vi "3 Totes Rotate.vi"() -> ()   [LabVIEW 2014]
panel:
  in  "Feet 4":dbl=6.0 format="%#_13g"
  in  "Degrees 2":dbl=45.0 format="%#_13g"
  in  "Feet 3":dbl=6.0 format="%#_13g"
  in  "Feet 2":dbl=6.0 format="%#_13g"
  in  "Degrees":dbl=45.0 format="%#_13g"
  in  "Feet":dbl=6.0 format="%#_13g"
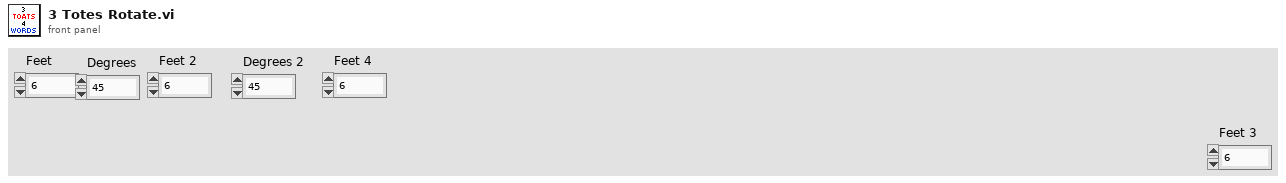
[diagram p1: front panel]
types:
  T1 = enum16{"Move Forward", "Move Backward", "Strafe Right", "Strafe Left"}
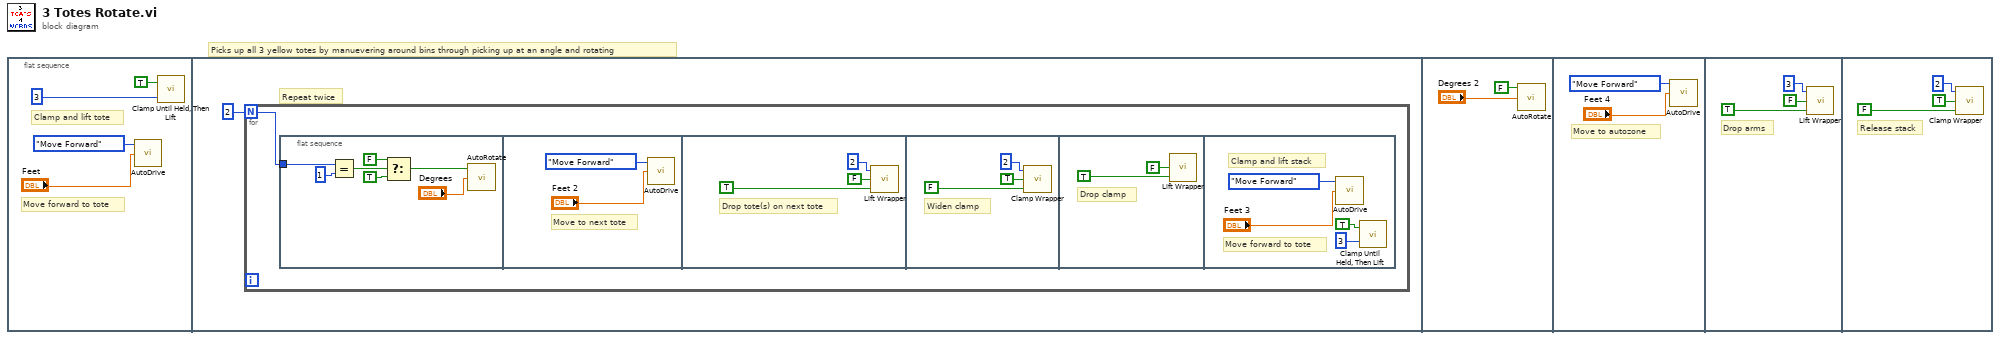
[diagram p0: block diagram]
diagram:
  # "Picks up all 3 yellow totes by manuevering around bins through picking up at an angle and rotating"
  n1 = flat-sequence {
    frame #0 {
      # "Clamp and lift tote"
      # "Move forward to tote"
      n2 = call "AutoDrive.vi"("Distance (ft)"="Feet", "Direction"=T1."Move Forward") -> ()  [unwired: 1 in, 1 out]
      n3 = call "Clamp Until Held, Then Lift.vi"("Iterations"=3, "Clamp + Lift"=TRUE) -> ()  [unwired: 1 in]
    }
    frame #1 {
      # "Repeat twice"
      n4 = for {
        N: 2 -> [w6]
        n5 = flat-sequence {
          tunnel: w6 -> [w12]
          frame #0 {
            n6 = Equal?(x=w12, y=1) -> (x = y?=w10:bool)
            n7 = Select(t=FALSE ("Clamp + Lift"), s=w10, f=TRUE ("Clamp + Lift")) -> (s? t:f=w7:bool)
            n8 = call "AutoRotate.vi"("Degrees"="Degrees", "Clockwise?"=w7) -> ()  [unwired: 1 in, 1 out]
          }
          frame #1 {
            # "Move to next tote"
            n9 = call "AutoDrive.vi"("Distance (ft)"="Feet 2", "Direction"=T1."Move Forward") -> ()  [unwired: 1 in, 1 out]
          }
          frame #2 {
            # "Drop tote(s) on next tote"
            n10 = call "Lift Wrapper.vi"("Down"=TRUE, "Up"=FALSE, "Iterations"=2) -> ()
          }
          frame #3 {
            # "Widen clamp"
            n11 = call "Clamp Wrapper.vi"("In"=FALSE ("In or Out"), "Out"=TRUE, "Iterations"=2) -> ()
          }
          frame #4 {
            # "Drop clamp"
            n12 = call "Lift Wrapper.vi"("Down"=TRUE ("Up or Down"), "Up"=FALSE) -> ()  [unwired: 1 in]
          }
          frame #5 {
            # "Move forward to tote"
            # "Clamp and lift stack"
            n13 = call "AutoDrive.vi"("Distance (ft)"="Feet 3", "Direction"=T1."Move Forward") -> ()  [unwired: 1 in, 1 out]
            n14 = call "Clamp Until Held, Then Lift.vi"("Iterations"=3, "Clamp + Lift"=TRUE) -> ()  [unwired: 1 in]
          }
        }
      }
    }
    frame #2 {
      n15 = call "AutoRotate.vi"("Degrees"="Degrees 2", "Clockwise?"=FALSE) -> ()  [unwired: 1 in, 1 out]
    }
    frame #3 {
      # "Move to autozone"
      n16 = call "AutoDrive.vi"("Distance (ft)"="Feet 4", "Direction"=T1."Move Forward") -> ()  [unwired: 1 in, 1 out]
    }
    frame #4 {
      # "Drop arms"
      n17 = call "Lift Wrapper.vi"("Down"=TRUE ("Up or Down"), "Up"=FALSE, "Iterations"=3) -> ()
    }
    frame #5 {
      # "Release stack"
      n18 = call "Clamp Wrapper.vi"("In"=FALSE ("In or Out"), "Out"=TRUE, "Iterations"=2) -> ()
    }
  }
